vi "Modules - Test Plan.vi"(8 "error in":errorcluster) -> (0 "error out":errorcluster)   [LabVIEW 2019]
uses:
  Controls/Test plan-state.ctl
  Controls/Test plan - Data Structure.ctl
  Controls/eFGV States.ctl
panel:
  in  "Tab Control":enum32{"Test Plans"}(tab)
  in  "table":i32(listbox)
  in  "Delete":bool
  in  "Edit":bool
  in  "New":bool
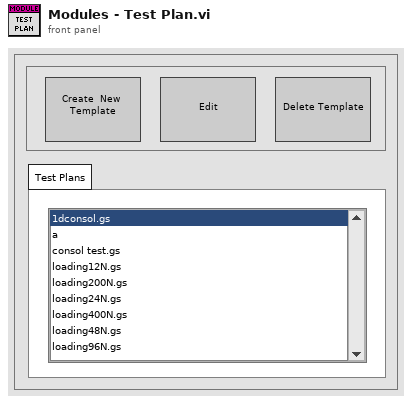
[diagram p1: front panel]
types:
  T1 = typedef "Test plan-state.ctl" = enum16{"Init", "Read", "Idle", "Edit", "Delete", "Close"}
  T2 = typedef "Test plan - Data Structure.ctl" = cluster{"Row":i32}
  T3 = enum32{"Invalid", "Standard", "Closed", "Hidden", "Minimized", "Maximized"}
  T4 = typedef "eFGV States.ctl" = enum16{"Init", "Read", "Write", "Exit"}
  T5 = typedef "Station - Test Type.ctl" = u16
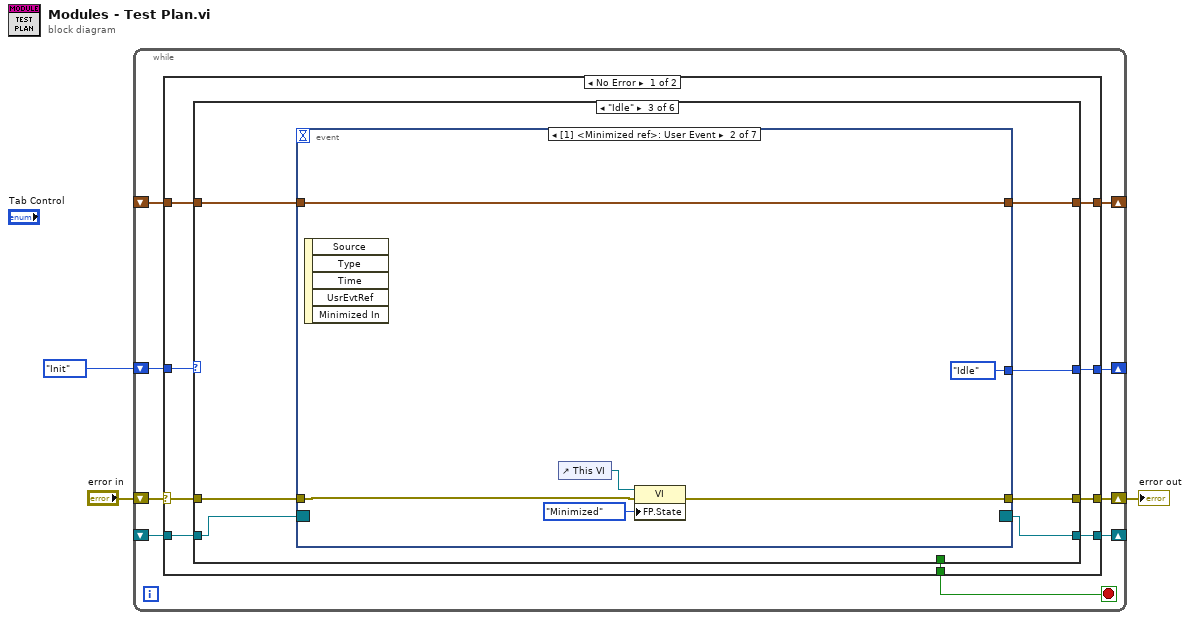
[diagram p0: block diagram]
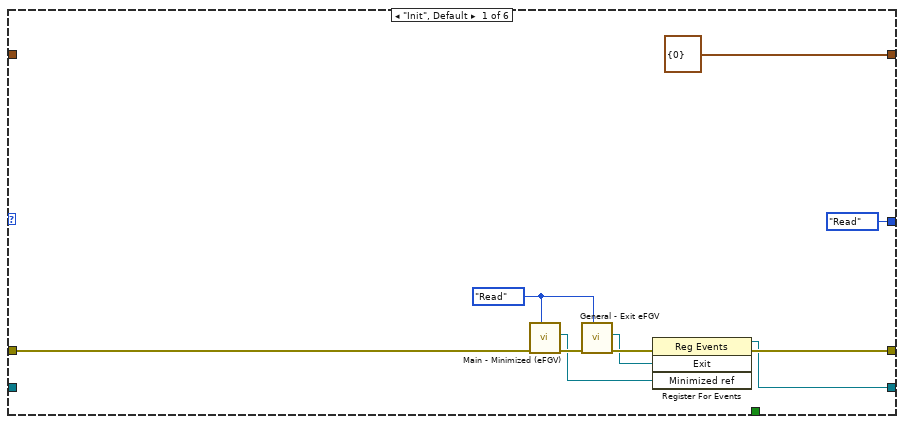
[diagram p2: hidden frame]
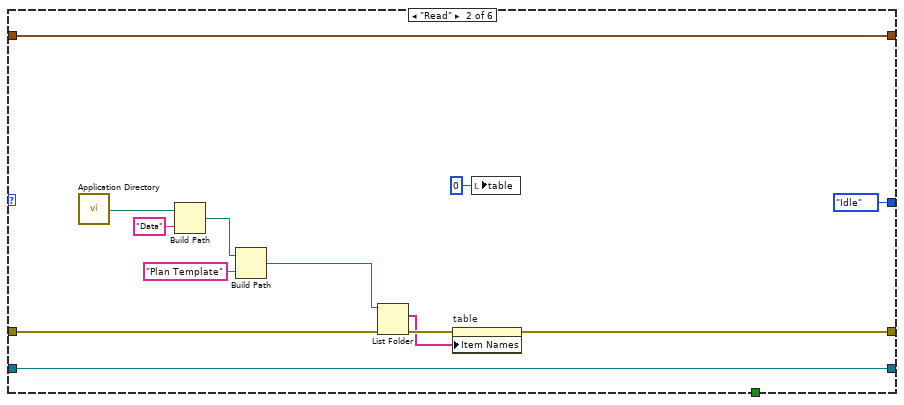
[diagram p3: hidden frame]
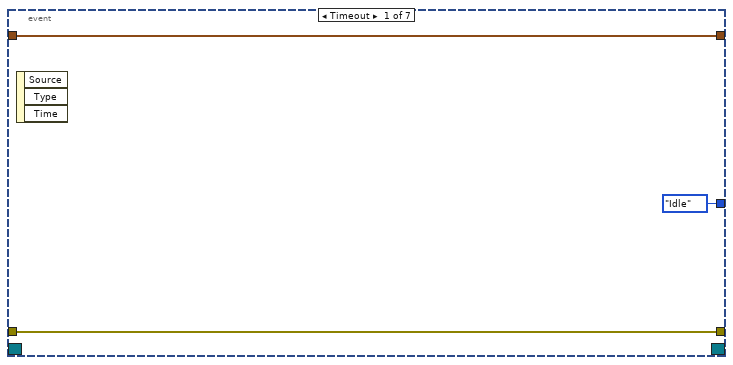
[diagram p4: hidden frame]
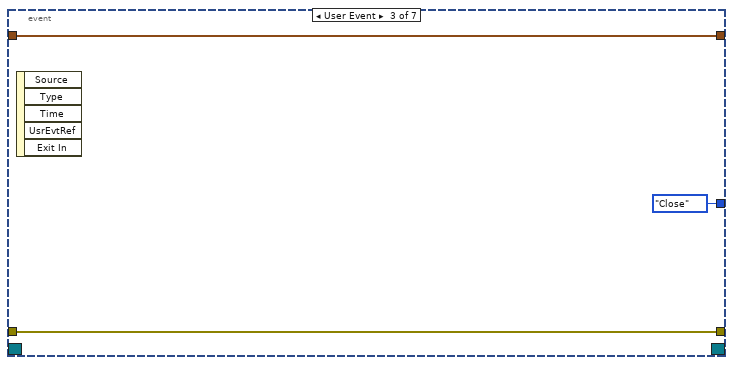
[diagram p5: hidden frame]
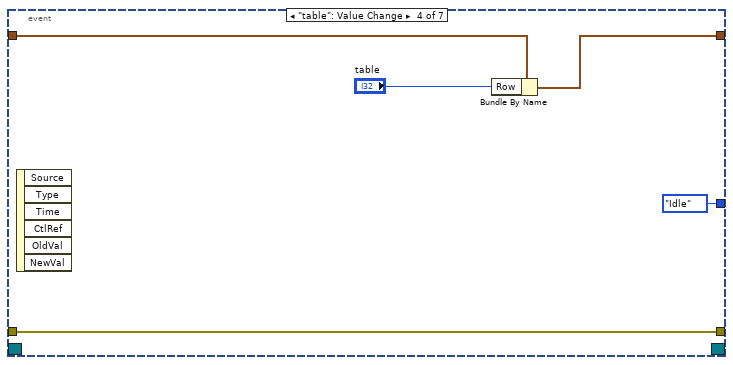
[diagram p6: hidden frame]
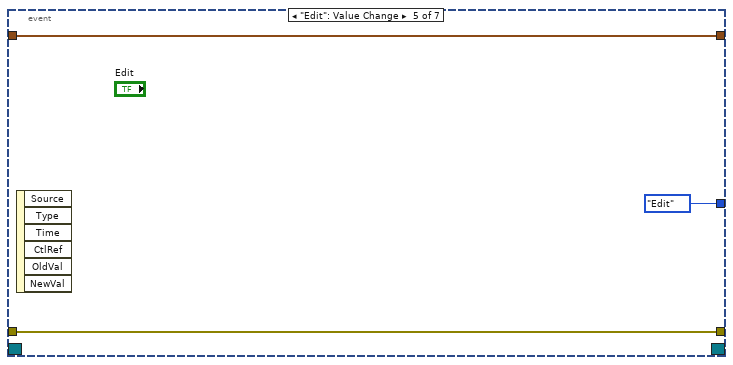
[diagram p7: hidden frame]
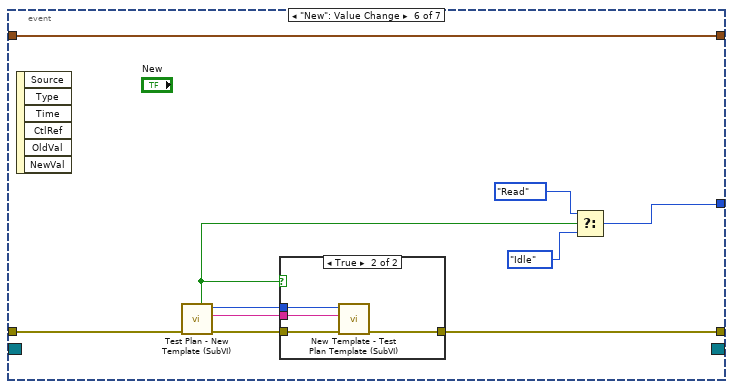
[diagram p8: hidden frame]
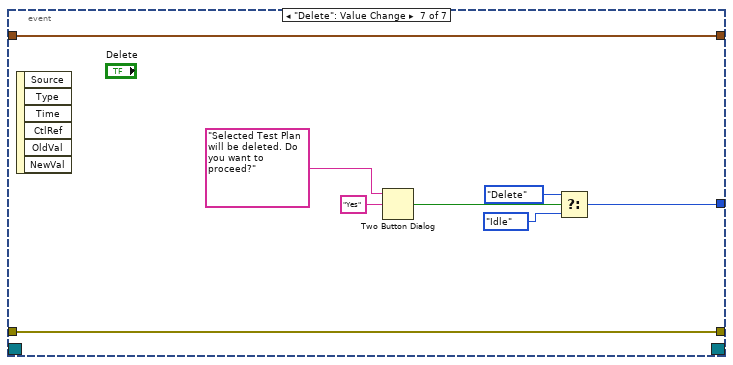
[diagram p10: hidden frame]
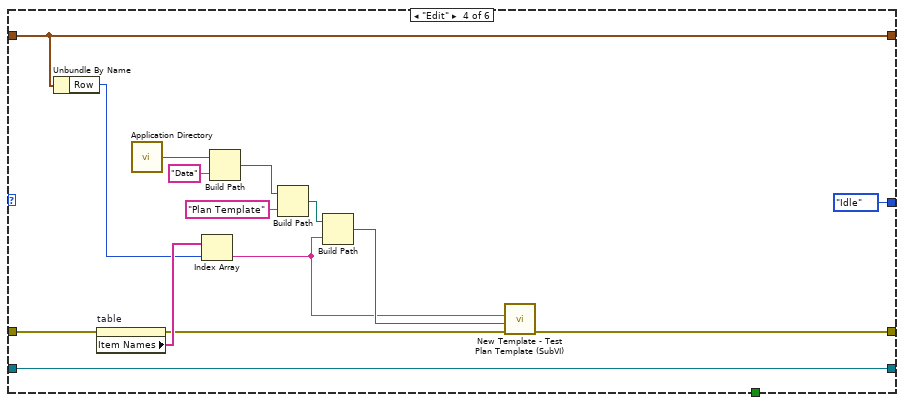
[diagram p11: hidden frame]
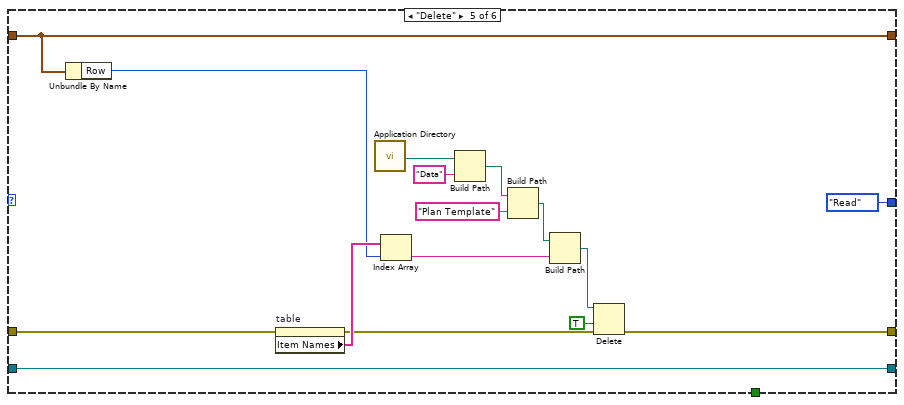
[diagram p12: hidden frame]
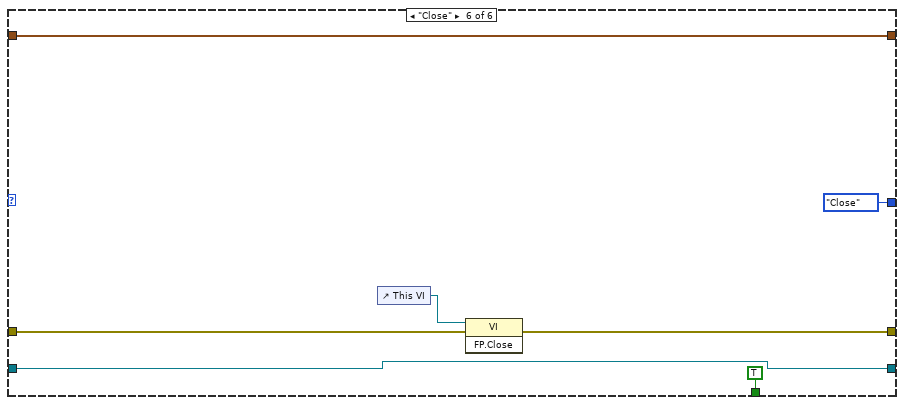
[diagram p13: hidden frame]
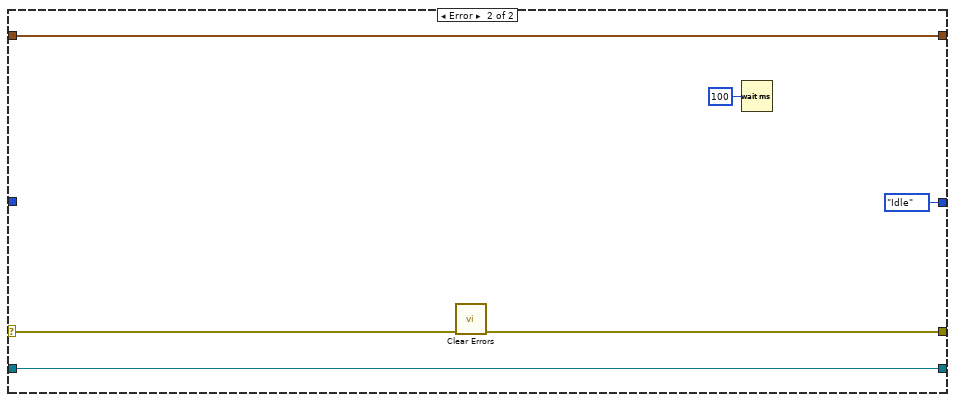
[diagram p14: hidden frame]
diagram:
  n1 = while {
    shift-right: [w8] -> w1
    shift-left: "error in" -> [w12]
    shift-right: [w10] -> _
    shift-left: Test_plan-state."Init" -> [w11]
    shift-right: [w7] -> _
    shift-left: _ -> [w6]
    shift-right: [w5] -> _
    shift-left: _ -> [w4]
    stop <- w9 stop-if-true
    n2 = case shown="No Error" w12 {
      selector: w12 -> [w19 w137]
      tunnel: w11 -> [w21 _]
      tunnel: [w20 Test_plan-state."Idle"] -> w10
      tunnel: [w18 _] -> w9
      tunnel: [w17 w134] -> w8
      tunnel: [w16 w138] -> w7
      tunnel: w6 -> [w15 w138]
      tunnel: [w14 w133] -> w5
      tunnel: w4 -> [w13 w133]
      frame No Error {
        n3 = case shown="\"Idle\"" w21 {
          tunnel: [Test_plan-state."Read" Test_plan-state."Idle" w47 Test_plan-state."Idle" Test_plan-state."Read" Test_plan-state."Close"] -> w20
          tunnel: w19 -> [w24 w43 w51 w105 w123 w127]
          tunnel: [_ _ _ _ _ TRUE ("T button?")] -> w18
          tunnel: [w28 w40 w50 w107 w116 w128] -> w17
          tunnel: [T2 {"Row"=0} w38 w49 w102 w122 w132] -> w16
          tunnel: w15 -> [_ w38 w48 w102 w122 w132]
          tunnel: [w26 w32 w45 w95 w110 w126] -> w14
          tunnel: w13 -> [_ w32 w46 w95 w110 w126]
          frame "Init", Default {
            w22 = eFGV_States."Read" ("eFGV States")
            n4 = call "Main - Minimized (eFGV).vi"("Action"=w22, "error in"=w24) -> ("error out"=w25:errorcluster, "Minimized ref"=w23:refnum<user-event>)  [unwired: 7 in, 1 out]
            n5 = call "General - Exit eFGV.vi"("eFGV States"=w22, "error in (no error)"=w25) -> ("error out"=w29:errorcluster, "Exit"=w27:refnum<user-event>)  [unwired: 7 in, 1 out]
            n6 = register-events(error in=w29, w27, w23) -> (reference out=w26:refnum<event-registration>, error out=w28:errorcluster)  [unwired: 1 in]
          }
          frame "Read" {
            n7 = call <vilib>:"Application Directory.vi"() -> ("Application Directory"=w34:path)
            n8 = Build Path(base path=w34, name or relative path="Data") -> (appended path=w33:path)
            n9 = Build Path(base path=w33, name or relative path="Plan Template") -> (appended path=w42:path)
            n10 = List Folder(path=w42, error in=w43) -> (filenames=w39:string[], error out=w41:errorcluster)  [unwired: 2 in, 2 out]
            n11 = property on="table" class="LstBox (strict)"(error in=w41, "Item Names"=w39) -> (error out=w40:errorcluster)  [unwired: 1 in, 1 out]
            n12 = local write "table"(0 ("table")) -> ()
          }
          frame "Idle" {
            n13 = event shown="[1] <Minimized ref>: User Event" {
              selector: w46 -> [_ _ _ _ _ _ _]
              dyn-events: [_ _ _ _ _ _ _] -> w45
              timeout: _ -> [_ _ _ _ _ _ _]
              tunnel: w51 -> [w54 w56 w63 w66 w71 w81 w92]
              tunnel: [w54 w55 w63 w66 w71 w75 w92] -> w50
              tunnel: [w53 w60 w62 w68 w70 w80 w91] -> w49
              tunnel: w48 -> [w53 w60 w62 w67 w70 w80 w91]
              tunnel: [Test_plan-state."Idle" Test_plan-state."Idle" Test_plan-state."Close" Test_plan-state."Idle" Test_plan-state."Edit" w78 w87] -> w47
              event Timeout {
                n14 = event-data() -> ()  [unwired: 1 in, 3 out]
              }
              event User Event {
                n15 = event-data() -> ()  [unwired: 1 in, 5 out]
                n16 = control-ref of="This VI"() -> (w58:refnum<vi>)
                n17 = property class="VI"(reference=w58, error in=w56, "FP.State"=T3."Minimized" ("Front Panel Window:State")) -> (error out=w55:errorcluster)  [unwired: 1 out]
              }
              event User Event {
                n18 = event-data() -> ()  [unwired: 1 in, 5 out]
              }
              event "table": Value Change {
                n19 = event-data() -> ()  [unwired: 1 in, 6 out]
                n20 = Bundle By Name(cluster=w67, "Row"="table") -> (w68:T2)
              }
              event "Edit": Value Change {
                n21 = event-data() -> ()  [unwired: 1 in, 6 out]
              }
              event "New": Value Change {
                n22 = event-data() -> ()  [unwired: 1 in, 6 out]
                n23 = call "Test Plan - New Template (SubVI).vi"("error in"=w81) -> ("error out"=w76:errorcluster, "Give a name for new Test Plan 2"=w73:string, "Test Type 2"=w74:T5, "save?"=w72:bool)  [unwired: 7 in]
                n24 = case shown="True" w72 {
                  tunnel: w76 -> [w82 w86]
                  tunnel: [w82 w85] -> w75
                  tunnel: w74 -> [_ w84]
                  tunnel: w73 -> [_ w83]
                  frame False {
                  }
                  frame True {
                    n25 = call "New Template - Test Plan Template (SubVI).vi"("error in"=w86, "File Name:"=w83, "Test Type"=w84) -> ("error out"=w85:errorcluster)  [unwired: 8 in]
                  }
                }
                n26 = Select(t=Test_plan-state."Read", s=w72, f=Test_plan-state."Idle") -> (s? t:f=w78:T1)
              }
              event "Delete": Value Change {
                n27 = event-data() -> ()  [unwired: 1 in, 6 out]
                n28 = Two Button Dialog(message="Selected Test Plan will be deleted. Do you want to proceed?", 2:"Yes" ("T button name (\"OK\")")) -> (T button?=w90:bool)  [unwired: 1 in]
                n29 = Select(t=Test_plan-state."Delete", s=w90, f=Test_plan-state."Idle") -> (s? t:f=w87:T1)
              }
            }
          }
          frame "Edit" {
            n30 = Unbundle By Name(w102) -> ("Row"=w101:i32)
            n31 = property on="table" class="LstBox (strict)"(error in=w105) -> (error out=w97:errorcluster, "Item Names"=w106:string[])  [unwired: 1 in, 1 out]
            n32 = call <vilib>:"Application Directory.vi"() -> ("Application Directory"=w99:path)
            n33 = Index Array(array=w106, index=w101) -> (element=w96:string)
            n34 = Build Path(base path=w99, name or relative path="Data") -> (appended path=w98:path)
            n35 = Build Path(base path=w98, name or relative path="Plan Template") -> (appended path=w104:path)
            n36 = Build Path(base path=w104, name or relative path=w96) -> (appended path=w103:path)
            n37 = call "New Template - Test Plan Template (SubVI).vi"("error in"=w97, "Load path"=w103, "File Name:"=w96) -> ("error out"=w107:errorcluster)  [unwired: 8 in]
          }
          frame "Delete" {
            n38 = Unbundle By Name(w122) -> ("Row"=w120:i32)
            n39 = property on="table" class="LstBox (strict)"(error in=w123) -> (error out=w117:errorcluster, "Item Names"=w121:string[])  [unwired: 1 in, 1 out]
            n40 = call <vilib>:"Application Directory.vi"() -> ("Application Directory"=w112:path)
            n41 = Index Array(array=w121, index=w120) -> (element=w118:string)
            n42 = Build Path(base path=w112, name or relative path="Data") -> (appended path=w111:path)
            n43 = Build Path(base path=w111, name or relative path="Plan Template") -> (appended path=w119:path)
            n44 = Build Path(base path=w119, name or relative path=w118) -> (appended path=w115:path)
            n45 = Delete(path (use dialog)=w115, confirm (F)=TRUE, error in=w117) -> (error out=w116:errorcluster)  [unwired: 2 in, 2 out]
          }
          frame "Close" {
            n46 = control-ref of="This VI"() -> (w129:refnum<vi>)
            n47 = invoke class="VI" method="FP.Close"(reference=w129, error in=w127) -> (error out=w128:errorcluster)  [unwired: 1 in, 2 out]
          }
        }
      }
      frame Error {
        n48 = call <vilib>:"Clear Errors.vi"("error in (no error)"=w137) -> ("error out"=w134:errorcluster)  [unwired: 5 in, 1 out]
        n49 = Wait (ms)(milliseconds to wait=u32 100) -> ()  [unwired: 1 out]
      }
    }
  }
  "error out" <- w1
